vi "map channels together.vi"(6 "owner 2":string, 7 "owner 1":string, 8 "error in":errorcluster, 9 "channel 2":refnum<class "TBM channel.lvclass">, 10 "channel 1":refnum<class "TBM channel.lvclass">, 11 "engine configuration":refnum<class "engine configuration.lvclass">) -> (0 "error out":errorcluster, 3 "engine configuration out":refnum<class "engine configuration.lvclass">)   [LabVIEW 2014, in "engine configuration.lvclass"]
doc: "This function maps two channels together. If types and classifications are compatible, and both channels are not currently mapped, this function will use either the single tag mapped to one of the channels or wil create a new tag from whichever channel is classified as a writer."
uses:
  engine configuration.lvclass
  <vilib>/NI/Tag Bus Module Framework/channel/TBM channel.lvclass
  <vilib>/NI/Tag Bus/tag/tag descriptor.lvclass/tag descriptor.ctl
  <vilib>/NI/Tag Bus Module Framework/channel/TBM channel.lvclass/TBM channel.ctl
  <vilib>/NI/Tag Bus Module Framework/channel/channel classification.ctl
  <vilib>/NI/Tag Bus/tag/tag descriptor.lvclass
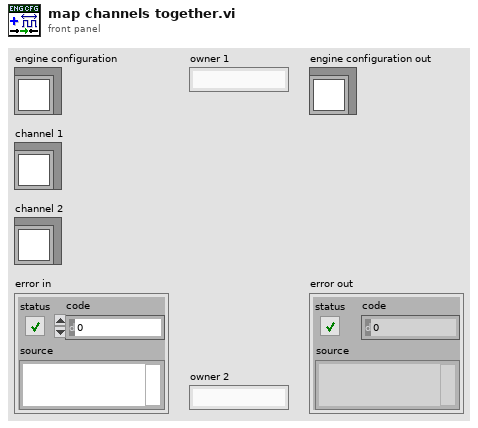
[diagram p1: front panel]
types:
  T1 = typedef "TBM channel.lvclass/channel classification.ctl" = enum16{"input data", "output data", "processing parameter", "processing result"}
  T2 = typedef "tag bus.lvlib/tag descriptor.lvclass/Data Type.ctl" = enum16{"Double", "Single", "I64", "I32", "I16", "I8", "U64", "U32", "U16", "U8", "Boolean", "String", "Array of Double", "Array of Single", "Array of I64", "Array of I32", "Array of I16", "Array of I8", "Array of U64", "Array of U32", "Array of U16", "Array of U8", "Array of Boolean", "Array of String"}
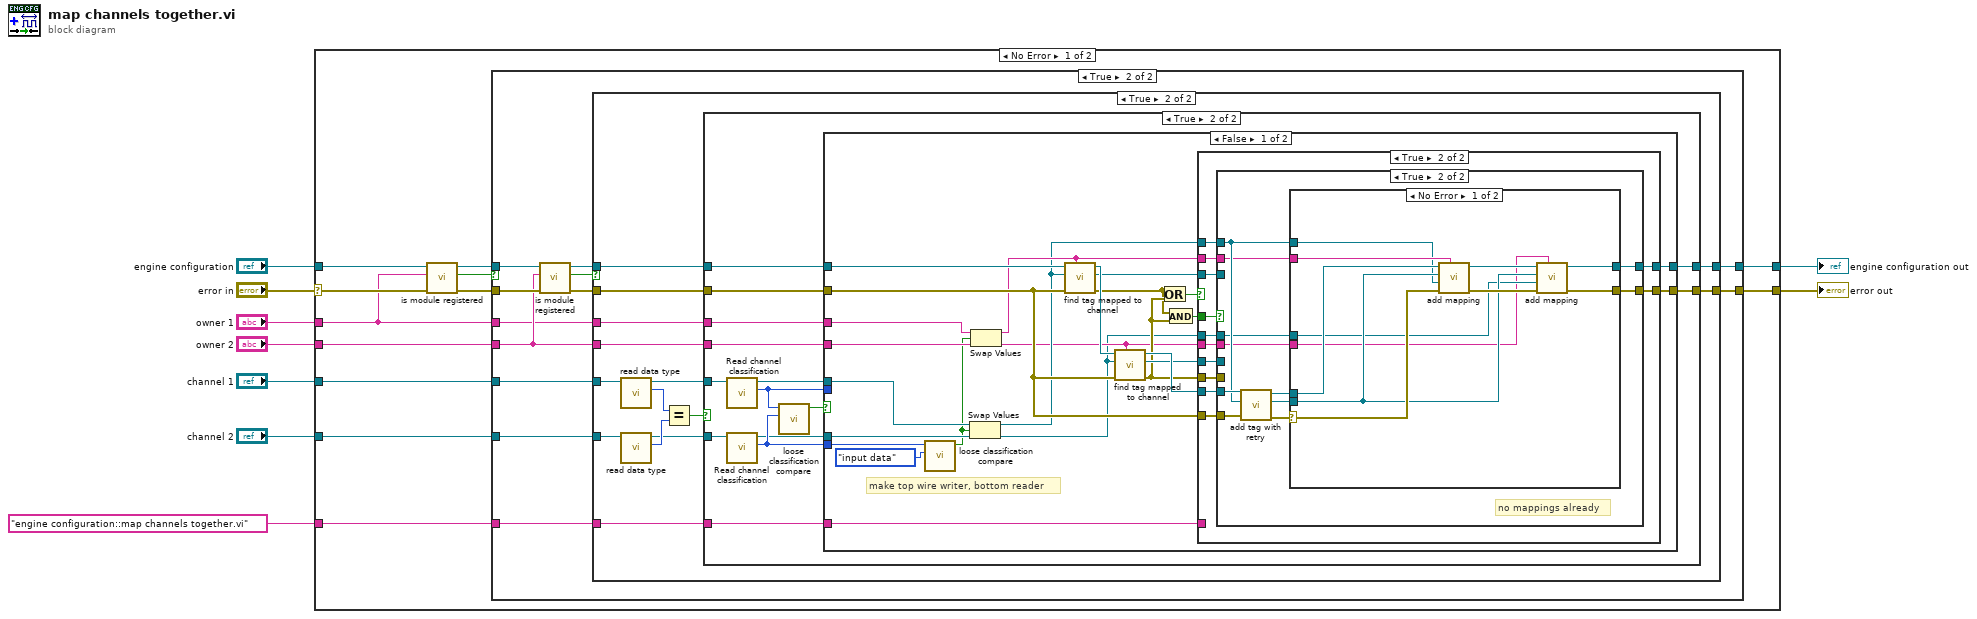
[diagram p0: block diagram]
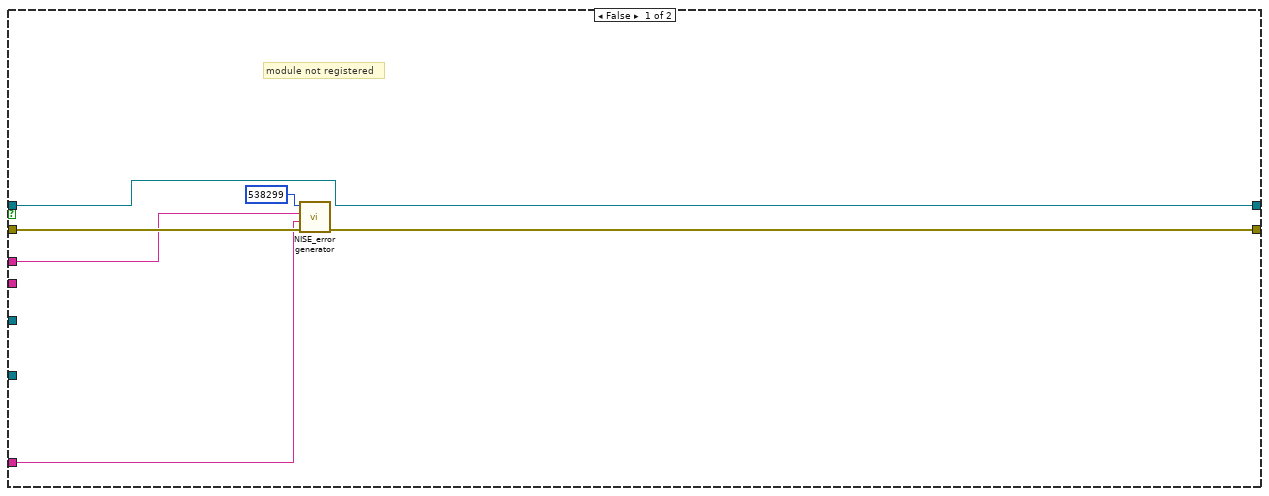
[diagram p2: hidden frame]
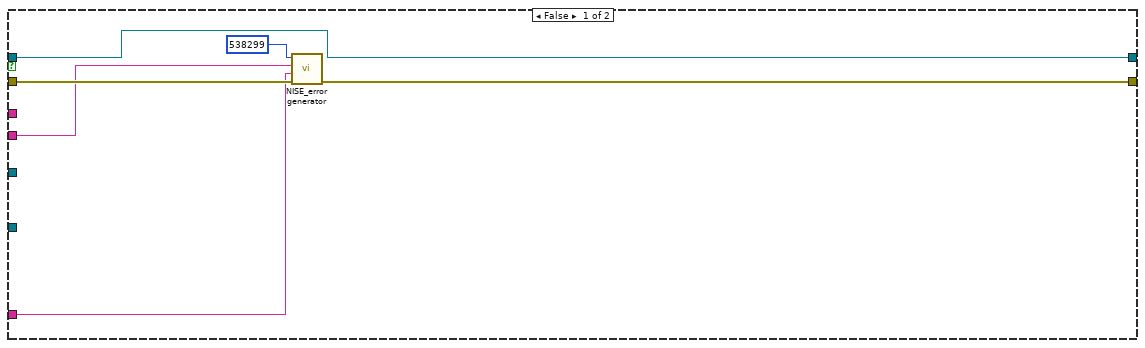
[diagram p3: hidden frame]
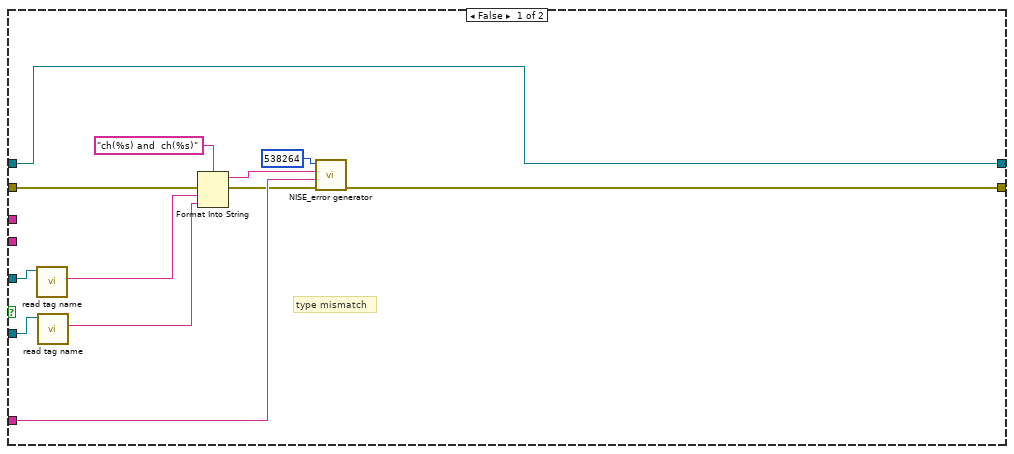
[diagram p4: hidden frame]
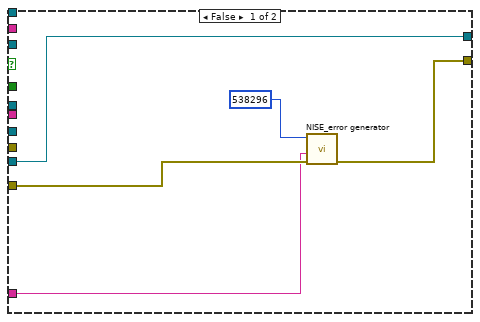
[diagram p5: hidden frame]
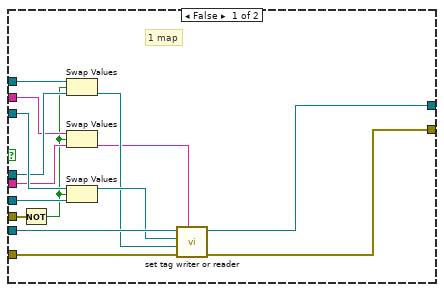
[diagram p6: hidden frame]
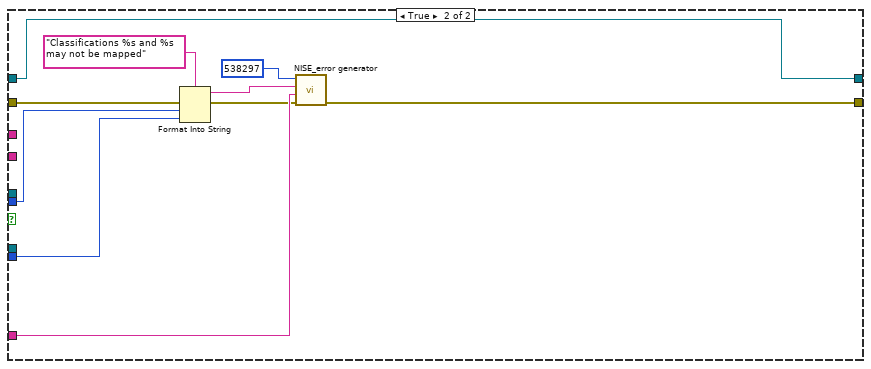
[diagram p8: hidden frame]
diagram:
  n1 = case shown="No Error" "error in" {
    selector: "error in" -> [w20 w177]
    tunnel: [w12 w177] -> w8
    tunnel: [w18 w176] -> w7
    tunnel: "engine configuration" -> [w21 w176]
    tunnel: "owner 1" -> [w13 _]
    tunnel: "owner 2" -> [w16 _]
    tunnel: "engine configuration::map channels together.vi" ("source") -> [w14 _]
    tunnel: "channel 1" -> [w11 _]
    tunnel: "channel 2" -> [w10 _]
    frame No Error {
      n2 = call-dynamic "is module registered.vi"("error in"=w20, "module ID"=w13, "engine configuration in"=w21) -> ("error out"=w17:errorcluster, "registered?"=w15:bool, "engine configuration out"=w19:refnum<class "engine configuration.lvclass">)  [unwired: 6 in]
      n3 = case shown="True" w15 {
        tunnel: w19 -> [w22 w39]
        tunnel: [w22 w35] -> w18
        tunnel: w17 -> [w26 w38]
        tunnel: w16 -> [_ w32]
        tunnel: w14 -> [w25 w33]
        tunnel: w13 -> [w24 w29]
        tunnel: [w23 w31] -> w12
        tunnel: w11 -> [_ w30]
        tunnel: w10 -> [_ w28]
        frame False {
          # "module not registered"
          n4 = call <vilib>:"NISE_error generator.vi"("error in"=w26, "source"=w25, "append error message"=w24, "error code (0)"=538299) -> ("error out"=w23:errorcluster)  [unwired: 5 in]
        }
        frame True {
          n5 = call-dynamic "is module registered.vi"("error in"=w38, "module ID"=w32, "engine configuration in"=w39) -> ("error out"=w34:errorcluster, "registered?"=w37:bool, "engine configuration out"=w36:refnum<class "engine configuration.lvclass">)  [unwired: 6 in]
          n6 = case shown="True" w37 {
            tunnel: w36 -> [w40 w54]
            tunnel: [w40 w48] -> w35
            tunnel: w34 -> [w44 w53]
            tunnel: w33 -> [w43 w52]
            tunnel: w32 -> [w42 w46]
            tunnel: [w41 w51] -> w31
            tunnel: w30 -> [_ w59]
            tunnel: w29 -> [_ w47]
            tunnel: w28 -> [_ w58]
            frame False {
              n7 = call <vilib>:"NISE_error generator.vi"("error in"=w44, "source"=w43, "append error message"=w42, "error code (0)"=538299) -> ("error out"=w41:errorcluster)  [unwired: 5 in]
            }
            frame True {
              n8 = call <vilib>:"read data type.vi"("system tag in"=w59) -> ("data type"=w56:T2, "system tag out"=w50:refnum<class "TBM channel.lvclass">)  [unwired: 8 in, 1 out]
              n9 = call <vilib>:"read data type.vi"("system tag in"=w58) -> ("data type"=w57:T2, "system tag out"=w49:refnum<class "TBM channel.lvclass">)  [unwired: 8 in, 1 out]
              n10 = Equal?(x=w56, y=w57) -> (x = y?=w55:bool)
              n11 = case shown="True" w55 {
                tunnel: w54 -> [w65 w79]
                tunnel: w53 -> [w70 w82]
                tunnel: w52 -> [w69 w81]
                tunnel: [w68 w80] -> w51
                tunnel: w50 -> [w67 w85]
                tunnel: w49 -> [w66 w84]
                tunnel: [w65 w78] -> w48
                tunnel: w47 -> [_ w73]
                tunnel: w46 -> [_ w72]
                frame False {
                  # "type mismatch"
                  n12 = call <vilib>:"read tag name.vi"("system tag in"=w67) -> ("name"=w61:string)  [unwired: 8 in, 2 out]
                  n13 = call <vilib>:"read tag name.vi"("system tag in"=w66) -> ("name"=w62:string)  [unwired: 8 in, 2 out]
                  n14 = Format Into String(format string="ch(%s) and  ch(%s)", error in=w70, w61, w62) -> (resulting string=w63:string, error out=w64:errorcluster)  [unwired: 1 in]
                  n15 = call <vilib>:"NISE_error generator.vi"("error in"=w64, "source"=w69, "append error message"=w63, "error code (0)"=538264) -> ("error out"=w68:errorcluster)  [unwired: 5 in]
                }
                frame True {
                  n16 = call <vilib>:"Read channel classification.vi"("channel in"=w85) -> ("channel classification"=w74:T1, "channel out"=w75:refnum<class "TBM channel.lvclass">)  [unwired: 8 in, 1 out]
                  n17 = call <vilib>:"Read channel classification.vi"("channel in"=w84) -> ("channel classification"=w77:T1, "channel out"=w76:refnum<class "TBM channel.lvclass">)  [unwired: 8 in, 1 out]
                  n18 = call "loose classification compare.vi"("class 2"=w77, "class 1"=w74) -> ("match?"=w83:bool)  [unwired: 9 in]
                  n19 = case shown="False" w83 {
                    tunnel: w82 -> [w99 w175]
                    tunnel: w81 -> [w96 w173]
                    tunnel: [w97 w172] -> w80
                    tunnel: w79 -> [w102 w171]
                    tunnel: [w98 w171] -> w78
                    tunnel: w77 -> [w108 w168]
                    tunnel: w76 -> [w107 _]
                    tunnel: w75 -> [w106 _]
                    tunnel: w74 -> [_ w167]
                    tunnel: w73 -> [w104 _]
                    tunnel: w72 -> [w105 _]
                    frame False {
                      # "make top wire writer, bottom reader"
                      n20 = call "loose classification compare.vi"("class 2"=channel_classification."input data", "class 1"=w108) -> ("match?"=w103:bool)  [unwired: 9 in]
                      n21 = Swap Values(12:w106, 13:w103, 14:w107) -> (1:w88:refnum<class "TBM channel.lvclass">, 3:w86:refnum<class "TBM channel.lvclass">)
                      n22 = Swap Values(12:w104, 13:w103, 14:w105) -> (1:w89:string, 3:w87:string)
                      n23 = call "find tag mapped to channel.vi"("owner"=w89, "error in"=w99, "channel"=w88, "engine configuration in"=w102) -> ("error out"=w91:errorcluster, "tag"=w94:refnum<class "tag descriptor.lvclass">, "engine configuration out"=w101:refnum<class "engine configuration.lvclass">)  [unwired: 5 in]
                      n24 = call "find tag mapped to channel.vi"("owner"=w87, "error in"=w99, "channel"=w86, "engine configuration in"=w101) -> ("error out"=w92:errorcluster, "tag"=w95:refnum<class "tag descriptor.lvclass">, "engine configuration out"=w100:refnum<class "engine configuration.lvclass">)  [unwired: 5 in]
                      n25 = Or(x=w91, y=w92) -> (x .or. y?=w93:bool)
                      n26 = And(x=w91, y=w92) -> (x .and. y?=w90:bool)
                      n27 = case shown="True" w93 {
                        tunnel: w100 -> [w114 w122]
                        tunnel: w99 -> [w113 w121]
                        tunnel: [w114 w116] -> w98
                        tunnel: [w112 w115] -> w97
                        tunnel: w96 -> [w110 _]
                        tunnel: w95 -> [_ w126]
                        tunnel: w94 -> [_ w125]
                        tunnel: w92 -> [_ w124]
                        tunnel: w90 -> [_ w123]
                        tunnel: w89 -> [_ w120]
                        tunnel: w88 -> [_ w119]
                        tunnel: w87 -> [_ w118]
                        tunnel: w86 -> [_ w117]
                        frame False {
                          n28 = call <vilib>:"NISE_error generator.vi"("error in"=w113, "source"=w110, "error code (0)"=538296) -> ("error out"=w112:errorcluster)  [unwired: 6 in]
                        }
                        frame True {
                          n29 = case shown="True" w123 {
                            tunnel: w126 -> [w141 _]
                            tunnel: w125 -> [w140 _]
                            tunnel: w124 -> [w139 _]
                            tunnel: w122 -> [w132 w152]
                            tunnel: w121 -> [w133 w151]
                            tunnel: w120 -> [w136 w144]
                            tunnel: w119 -> [w135 w145]
                            tunnel: w118 -> [w138 w142]
                            tunnel: w117 -> [w137 w143]
                            tunnel: [w128 w148] -> w116
                            tunnel: [w127 w147] -> w115
                            frame False {
                              # "1 map"
                              n30 = Not(x=w139) -> (.not. x?=w134:bool)
                              n31 = Swap Values(12:w135, 13:w134, 14:w137) -> (3:w130:refnum<class "TBM channel.lvclass">)  [unwired: 1 out]
                              n32 = Swap Values(12:w136, 13:w134, 14:w138) -> (3:w129:string)  [unwired: 1 out]
                              n33 = Swap Values(12:w140, 13:w134, 14:w141) -> (1:w131:refnum<class "tag descriptor.lvclass">)  [unwired: 1 out]
                              n34 = call-dynamic "set tag writer or reader.vi"("module GUID"=w129, "error in"=w133, "channel"=w130, "tag descriptor"=w131, "engine configuration in"=w132) -> ("error out"=w127:errorcluster, "engine configuration out"=w128:refnum<class "engine configuration.lvclass">)  [unwired: 5 in]
                            }
                            frame True {
                              # "no mappings already"
                              n35 = call "add tag with retry.vi"("error in"=w151, "tag in"=w145, "engine configuration in"=w152) -> ("error out"=w150:errorcluster, "tag out"=w146:refnum<class "tag descriptor.lvclass">, "engine configuration out"=w149:refnum<class "engine configuration.lvclass">)  [unwired: 6 in]
                              n36 = case shown="No Error" w150 {
                                selector: w150 -> [w163 w164]
                                tunnel: w149 -> [w161 w165]
                                tunnel: [w158 w165] -> w148
                                tunnel: [w160 w164] -> w147
                                tunnel: w146 -> [w157 _]
                                tunnel: w145 -> [w153 _]
                                tunnel: w144 -> [w154 _]
                                tunnel: w143 -> [w156 _]
                                tunnel: w142 -> [w155 _]
                                frame No Error {
                                n37 = call-dynamic "add mapping.vi"("owner ID"=w154, "error in"=w163, "channel"=w153, "tag descriptor"=w157, "engine configuration"=w161) -> ("error out"=w162:errorcluster, "engine configuration out"=w159:refnum<class "engine configuration.lvclass">)  [unwired: 5 in]
                                n38 = call-dynamic "add mapping.vi"("owner ID"=w155, "error in"=w162, "channel"=w156, "tag descriptor"=w157, "engine configuration"=w159) -> ("error out"=w160:errorcluster, "engine configuration out"=w158:refnum<class "engine configuration.lvclass">)  [unwired: 5 in]
                                }
                                frame Error {
                                }
                              }
                            }
                          }
                        }
                      }
                    }
                    frame True {
                      n39 = Format Into String(format string="Classifications %s and %s may not be mapped", error in=w175, w167, w168) -> (resulting string=w169:string, error out=w170:errorcluster)  [unwired: 1 in]
                      n40 = call <vilib>:"NISE_error generator.vi"("error in"=w170, "source"=w173, "append error message"=w169, "error code (0)"=538297) -> ("error out"=w172:errorcluster)  [unwired: 5 in]
                    }
                  }
                }
              }
            }
          }
        }
      }
    }
    frame Error {
    }
  }
  "error out" <- w8
  "engine configuration out" <- w7
